vi "ReadScanPatternGen.vi"(4 "Error in":errorcluster, 5 "VarParam":string, 7 "Modèle":string) -> (0 "Error out":errorcluster, 1 "Positions":dbl[](array[numeric]) format="%#.2g", 3 "Modèles":string[](array[string]))   [LabVIEW 2019]
doc: "Ce VI ouvre le fichier de sauvegarde des modèles et lit les positions du modèle spécifié."
uses:
  <vilib>/Utility/config.llb/Read Key (String).vi
  <vilib>/Utility/config.llb/NI_LVConfig.lvlib
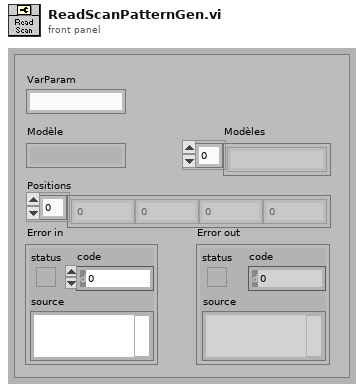
[diagram p1: front panel]
types:
  T1 = typedef "NI_LVConfig.lvlib/Config Data RefNum.ctl" = refnum<k1>
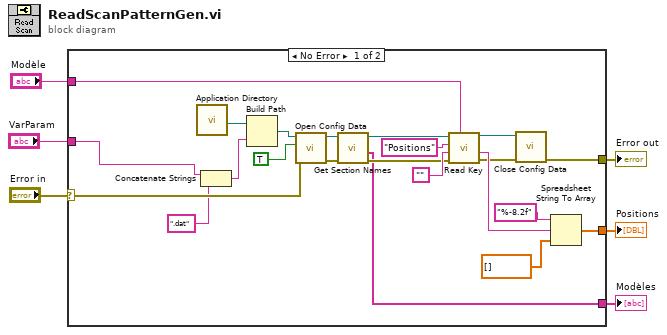
[diagram p0: block diagram]
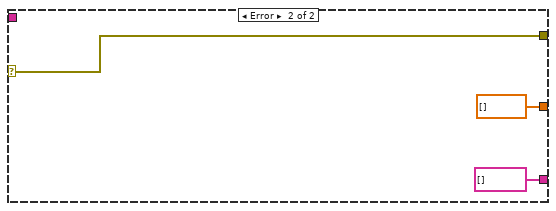
[diagram p2: hidden frame]
diagram:
  n1 = case shown="No Error" "Error in" {
    selector: "Error in" -> [w18 w31]
    tunnel: "Modèle" -> [w26 _]
    tunnel: [w22 dbl[] [] ("array type (2D Dbl)")] -> w5
    tunnel: [w19 w31] -> w4
    tunnel: [w13 string[] [] ("section names")] -> w2
    tunnel: "VarParam" -> [w8 _]
    frame No Error {
      n2 = call <vilib>:"Application Directory.vi"() -> ("Application Directory"=w7:path)
      n3 = Concatenate Strings(w8, ".dat" ("chaîne")) -> (w9:string)
      n4 = Build Path(base path=w7, name or relative path=w9) -> (appended path=w27:path)
      n5 = call <vilib>:"Open Config Data.vi"("error in (no error)"=w18, "create file if necessary (T)"=TRUE ("create file if necessary? (T)"), "configuration file path"=w27) -> ("error out"=w17:errorcluster, "refnum"=w16:T1)  [unwired: 6 in, 1 out]
      n6 = call <vilib>:"Get Section Names.vi"("error in (no error)"=w17, "refnum"=w16) -> ("error out"=w14:errorcluster, "section names"=w13:string[], "refnum out"=w15:T1)  [unwired: 7 in]
      n7 = call-poly <vilib>:"Read Key.vi"("section"=w26, "error in (no error)"=w14, "default value"="", "key"="Positions", "refnum"=w15) -> ("error out"=w12:errorcluster, "value"=w21:string, "refnum out"=w11:T1)  [unwired: 3 in, 1 out]
      n8 = call <vilib>:"Close Config Data.vi"("error in (no error)"=w12, "refnum"=w11) -> ("error out"=w19:errorcluster)  [unwired: 8 in, 1 out]
      n9 = Spreadsheet String To Array(format string="%-8.2f", spreadsheet string=w21, array type (2D Dbl)=dbl[] []) -> (array=w22:dbl[])  [unwired: 1 in]
    }
    frame Error {
    }
  }
  "Positions" <- w5
  "Error out" <- w4
  "Modèles" <- w2
